vi "SWITCH Message Loop.vi"(8 "error in (no error)":errorcluster) -> (0 "error out":errorcluster)   [LabVIEW 2020, in "MOTOR.lvlib"]
doc: "Message loop for handling messages pertaining to the acquisition of data from the hardware."
uses:
  MOTOR.lvlib
  support/PCT FGV CMD.ctl
  Acquisition State.ctl
  PS Hardware Configuration.ctl
  support/Message Queue/Message Cluster.ctl
  support/Message Queue/Enqueue Message (Single).vi
  <vilib>/Utility/error.llb/Error Cluster From Error Code.vi
  <vilib>/ErrorRing/Error Ring.xnode
  support/Message Queue/Message Queue.lvlib
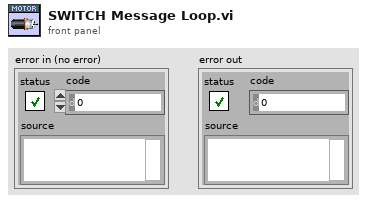
[diagram p1: front panel]
types:
  T1 = typedef "PCT FGV CMD.ctl" = enum16{"INIT", "GET", "SET"}
  T2 = typedef "Message Queue.lvlib/All Message Queues.ctl" = cluster{"UI":refnum<queue>, "Logging":refnum<queue>, "LOG":refnum<queue>, "ALARM":refnum<queue>, "Test":refnum<queue>, "Answer":refnum<queue>, "PLC":refnum<queue>, "DB":refnum<queue>, "Report":refnum<queue>, "OPC":refnum<queue>, "Procedure":refnum<queue>, "PalmSens":refnum<queue>, "SYS 7000 Reader":refnum<queue>, "SWITCH":refnum<queue>, "MOTOR":refnum<queue>, "MOTION":refnum<queue>, "HIDEN":refnum<queue>, "VALVE":refnum<queue>, "MFC":refnum<queue>, "PUMP IN":refnum<queue>, "PUMP OUT":refnum<queue>}
  T3 = typedef "PCT Data REFs.ctl" = cluster{"PLC AI Notifier":refnum<notifier>, "PS Data Queue":refnum<queue>, "BTN Queue":refnum<queue>, "PLC DI notifier":refnum<notifier>, "Timer notifier":refnum<notifier>, "DMM PS":refnum<notifier>, "DMM Gages":refnum<notifier>, "XYZ notifier":refnum<notifier>, "Test Notifier":refnum<notifier>, "Scanner notifier":refnum<notifier>, "OPC Notifier":refnum<notifier>, "HIDEN queue":refnum<queue>}
  T4 = typedef "MOTOR.lvlib/PS Hardware Configuration.ctl" = cluster{"Tango HW":cluster{"VISA resource":refnum<visa-resource-name>, "Baud Rate (115200)":i32, "lAnInterfaceType":i32, "bAShowProt":i32}, "Writer Queue":refnum<queue>, "Status":bool, "Abs Position":i32[], "Axis Velocity":cluster{"dX":dbl, "dY":dbl, "dZ":dbl, "dA":dbl}, "acceleration ":dbl, "Z direction":enum16{"Up", "Down"}, "Position Mode":string, "plLSID":i32}
  T5 = typedef "Message Queue.lvlib/Message Cluster.ctl" = cluster{"Message":string, "Message Data":variant}
  T6 = typedef "MOTOR.lvlib/Acquisition State.ctl" = enum16{"Idle", "Initialized"}
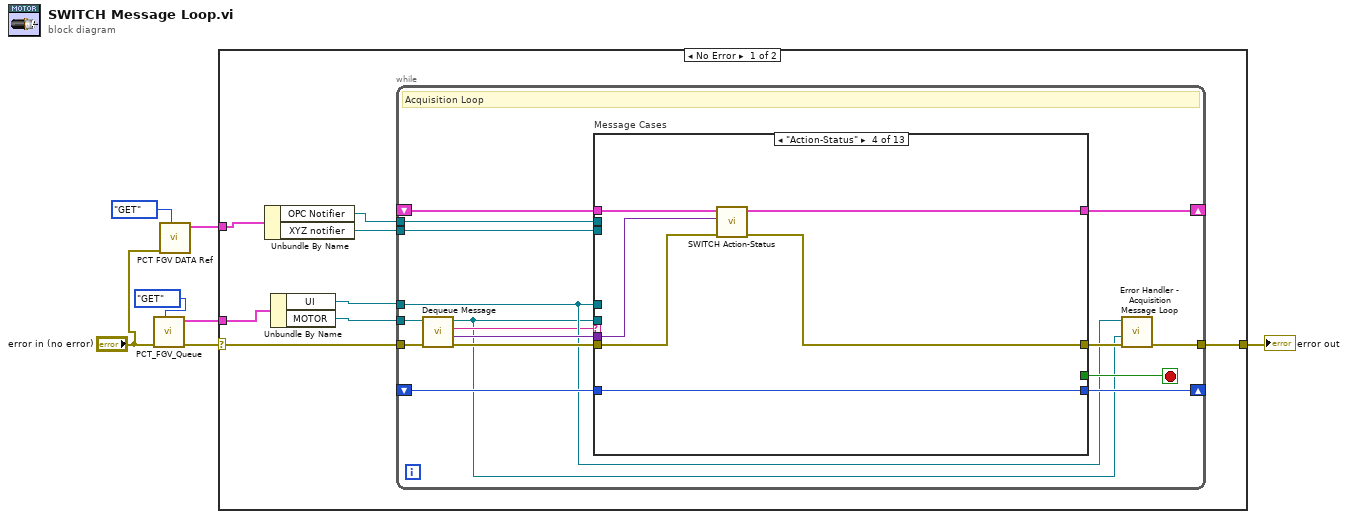
[diagram p0: block diagram]
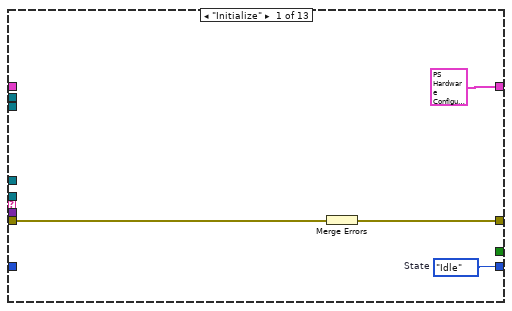
[diagram p2: hidden frame]
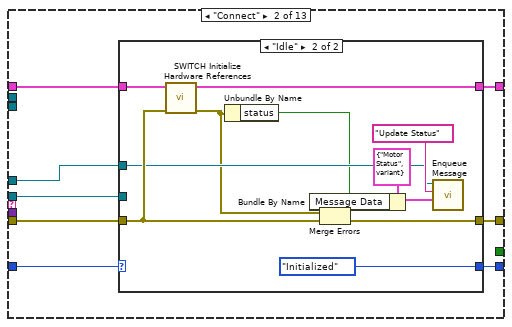
[diagram p3: hidden frame]
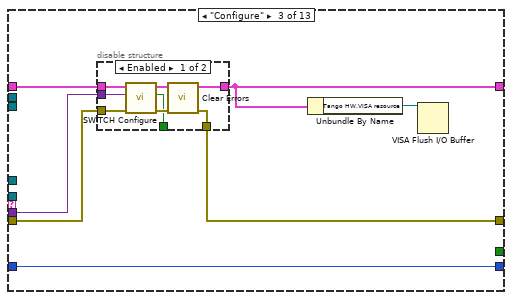
[diagram p5: hidden frame]
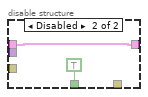
[diagram p6: hidden frame]
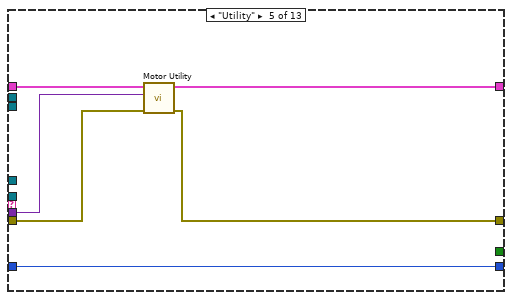
[diagram p7: hidden frame]
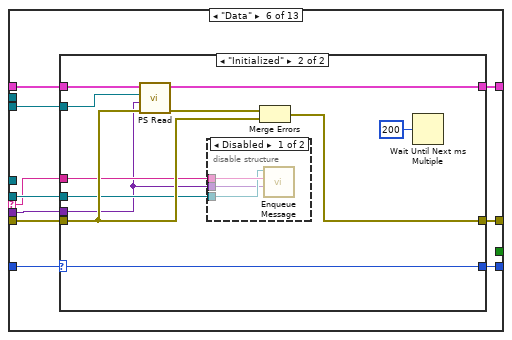
[diagram p8: hidden frame]
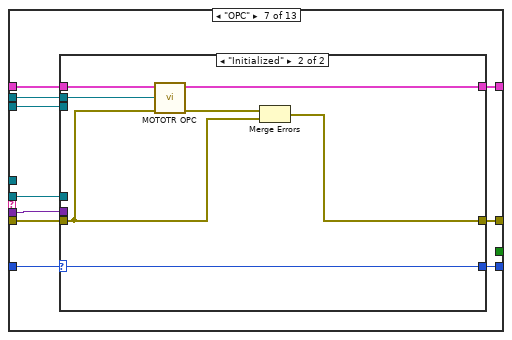
[diagram p11: hidden frame]
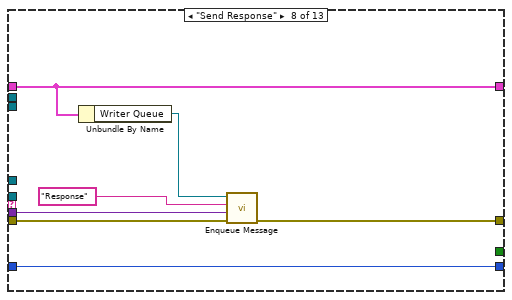
[diagram p13: hidden frame]
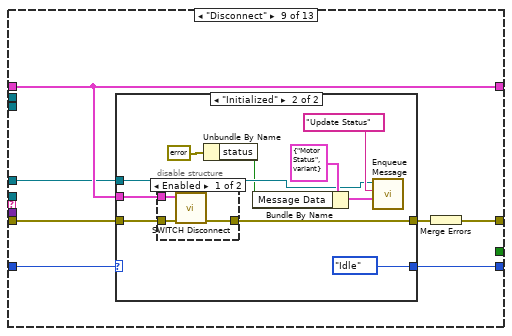
[diagram p14: hidden frame]
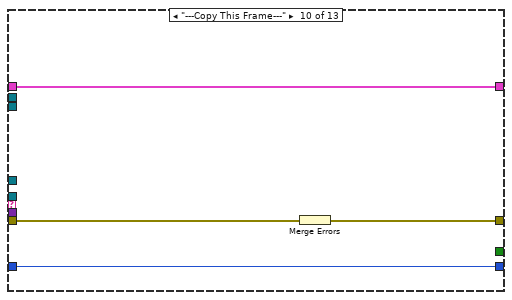
[diagram p17: hidden frame]
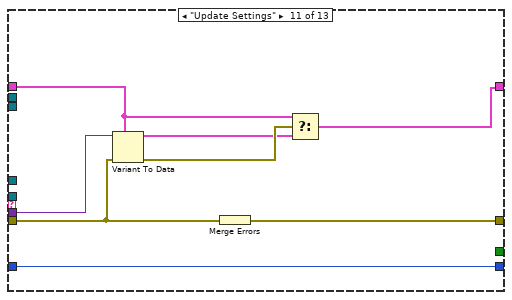
[diagram p18: hidden frame]
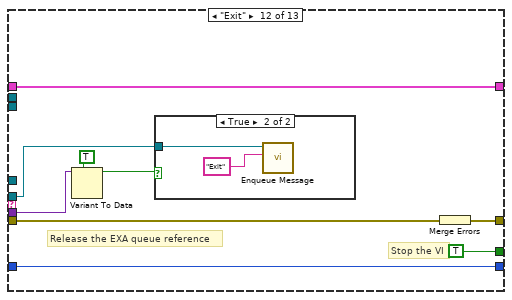
[diagram p19: hidden frame]
diagram:
  n1 = call "PCT_FGV_Queue.vi"("CMD"=PCT_FGV_CMD."GET", "error in (no error)"="error in (no error)") -> ("error out"=w5:errorcluster, "Message Queues out"=w4:T2)  [unwired: 8 in]
  n2 = call "PCT FGV DATA Ref.vi"("CMD"=PCT_FGV_CMD."GET", "error in (no error)"="error in (no error)") -> ("Data REF"=w1:T3)  [unwired: 8 in, 1 out]
  n3 = case shown="No Error" w5 {
    selector: w5 -> [w12 w196]
    tunnel: w4 -> [w15 _]
    tunnel: [w13 w196] -> w7
    tunnel: w1 -> [w10 _]
    frame No Error {
      n4 = Unbundle By Name(w10) -> ("OPC Notifier"=w8:refnum<notifier>, "XYZ notifier"=w9:refnum<notifier>)
      n5 = Unbundle By Name(w15) -> ("UI"=w11:refnum<queue>, "MOTOR"=w14:refnum<queue>)
      n6 = while {
        tunnel: w14 -> [w25]
        shift-right: [w30] -> _
        shift-left: _ -> [w31]
        tunnel: w11 -> [w20]
        shift-right: [w23] -> _
        shift-left: _ -> [w24]
        tunnel: w12 -> [w28]
        tunnel: [w22] -> w13
        tunnel: w9 -> [w18]
        tunnel: w8 -> [w16]
        stop <- w29 stop-if-true
        # "Acquisition Loop"
        n7 = call "Dequeue Message.vi"("error in (no error)"=w28, "Message Queue"=w25) -> ("error out"=w27:errorcluster, "Message Data"=w26:variant, "Message"=w19:string, "dup Message Queue"=w17:refnum<queue>)  [unwired: 6 in]
        n8 = case "Message Cases" shown="\"Action-Status\"" w19 {
          selector: w19 -> [_ _ _ _ _ w86 _ _ _ _ _ _ w185]
          tunnel: w17 -> [_ w40 _ _ _ w94 w121 _ _ _ _ w176 _]
          tunnel: w27 -> [w34 w41 w61 w75 w82 w93 w120 w137 w145 w165 w167 w175 _]
          tunnel: [w35 w43 w60 w74 w80 w95 w122 w136 w146 w163 w173 w181 w186] -> w21
          tunnel: w31 -> [_ w42 w62 w76 w84 w91 w118 w134 w143 w164 w169 w180 w188]
          tunnel: [T4 {"Tango HW"={"VISA resource"="", "Baud Rate (115200)"=0, "lAnInterfaceType"=0, "bAShowProt"=2}, "Writer Queue"=refnum, "Status"=FALSE, "Abs Position"=[], "Axis Velocity"={"dX"=0.0, "dY"=0.0, "dZ"=0.0, "dA"=0.0}, "acceleration "=0.0, "Z direction"=enum."Up", "Position Mode"="", "plLSID"=0} ("Data Cluster") w39 w59 w77 w81 w92 w119 w134 w143 w164 w168 w180 w188] -> w30
          tunnel: [_ _ _ _ _ _ _ _ _ _ _ TRUE _] -> w29
          tunnel: w26 -> [_ _ w63 w78 w83 w88 w115 w135 _ _ w172 w174 _]
          tunnel: w20 -> [_ w36 _ _ _ _ _ _ w140 _ _ _ _]
          tunnel: w24 -> [_ w37 w64 w79 w85 w89 w116 w138 w142 w162 w166 w179 w187]
          tunnel: [w33 w38 w64 w79 w85 w90 w117 w138 w141 w162 w166 w179 w187] -> w23
          tunnel: w18 -> [_ _ _ _ _ w87 w114 _ _ _ _ _ _]
          tunnel: w16 -> [_ _ _ _ _ _ w113 _ _ _ _ _ _]
          frame "Initialize" {
            w33 = Acquisition_State."Idle"  # State
            # "Initialize  - Initialize is currently a no-op.  The hardware initialization takes place in the 'Start' message."
            n9 = Merge Errors(w34) -> (w35:errorcluster)
          }
          frame "Connect" {
            # "Start - Configure and start the acquisition."
            n10 = case shown="\"Idle\"" w37 {
              selector: w37 -> [w44 _]
              tunnel: [w45 w57] -> w43
              tunnel: w42 -> [w46 w56]
              tunnel: w41 -> [w45 w53]
              tunnel: w40 -> [_ _]
              tunnel: [w46 w55] -> w39
              tunnel: [w44 Acquisition_State."Initialized" ("Acquisition State")] -> w38
              tunnel: w36 -> [_ w49]
              frame "Initialized" {
                # "The system is already acquiring. Ignore the \"Start\" message."
              }
              frame "Idle" {
                # "If the system is idle, start the acquisition."
                n11 = call "SWITCH Initialize Hardware References.vi"("error in (no error)"=w53, "Hardware Resources in"=w56) -> ("error out"=w48:errorcluster, "Hardware Resources out"=w55:T4)  [unwired: 8 in]
                n12 = Unbundle By Name(w48) -> ("status"=w47:bool)
                n13 = Bundle By Name(cluster=T5 {"Message"="Motor Status", "Message Data"=variant} ("Message Cluster"), "Message Data"=w47) -> (w51:T5)
                n14 = Merge Errors(w48, w53) -> (w57:errorcluster)
                n15 = call-poly "Enqueue Message.vi"("Message Data"=w51, "Message"="Update Status", "Message Queue"=w49) -> ()  [unwired: 7 in, 2 out]
              }
            }
          }
          frame "Configure" {
            # "Start - Configure and start the acquisition."
            n16 = disable-structure shown="Enabled" {
              disable-tunnel: w63 -> [w71 _]
              disable-tunnel: w62 -> [w70 w73]
              disable-tunnel: w61 -> [w69 _]
              disable-tunnel: [w67 w73] -> w59
              disable-tunnel: [w66 _] -> w60
              disable-tunnel: [w65 TRUE ("Send Resp")] -> _
              frame Enabled {
                n17 = call "SWITCH Configure.vi"("error in (no error)"=w69, "Message Data"=w71, "Data Cluster"=w70) -> ("error out"=w68:errorcluster, "Send Resp"=w65:bool, "Data Cluster out"=w67:T4)  [unwired: 6 in]
                n18 = call <vilib>:"Clear Errors.vi"("error in (no error)"=w68) -> ("error out"=w66:errorcluster)  [unwired: 5 in, 1 out]
              }
              frame Disabled {
              }
            }
            n19 = Unbundle By Name(w59) -> ("Tango HW.VISA resource"=w58:refnum<visa-resource-name>)
            n20 = VISA Flush I/O Buffer(VISA resource name=w58) -> ()  [unwired: 2 in, 2 out]
          }
          frame "Action-Status" {
            # "Start - Configure and start the acquisition."
            n21 = call "SWITCH Action-Status.vi"("error in (no error)"=w75, "Message Data"=w78, "Data Cluster"=w76) -> ("error out"=w74:errorcluster, "Data Cluster out"=w77:T4)  [unwired: 7 in]
          }
          frame "Utility" {
            # "Start - Configure and start the acquisition."
            n22 = call "Motor Utility.vi"("error in (no error)"=w82, "Message Data"=w83, "Data Cluster"=w84) -> ("error out"=w80:errorcluster, "Data Cluster out"=w81:T4)  [unwired: 7 in]
          }
          frame "Data" {
            # "Acquire - Acquire data from the hardware. Since this is a continuous acquisition, this message will always message itself to run again."
            n23 = case shown="\"Initialized\"" w89 {
              selector: w89 -> [w96 w105]
              tunnel: [w97 w109] -> w95
              tunnel: w94 -> [_ w101]
              tunnel: w93 -> [w97 w103]
              tunnel: [w98 w107] -> w92
              tunnel: w91 -> [w98 w106]
              tunnel: [w96 w105] -> w90
              tunnel: w88 -> [_ w99]
              tunnel: w87 -> [_ w104]
              tunnel: w86 -> [_ w102]
              frame "Idle" {
              }
              frame "Initialized" {
                # "Read  data"
                n24 = call "PS Read.vi"("error in (no error)"=w103, "Message Data"=w99, "XYZ notifier"=w104, "Hardware Resources in"=w106) -> ("error out"=w108:errorcluster, "Hardware Resources out"=w107:T4)  [unwired: 5 in, 1 out]
                n25 = disable-structure shown="Disabled" {
                  disable-tunnel: w102 -> [w112 _]
                  disable-tunnel: w101 -> [w111 _]
                  disable-tunnel: w99 -> [w110 _]
                  frame Disabled {
                    n26 = call-poly "Enqueue Message.vi"("Message Data"=w110, "Message"=w112, "Message Queue"=w111) -> ()  [unwired: 7 in, 2 out]
                  }
                  frame Enabled {
                  }
                }
                n27 = Merge Errors(w108, w103) -> (w109:errorcluster)
                n28 = Wait Until Next ms Multiple(millisecond multiple=u32 200) -> ()  [unwired: 1 out]
              }
            }
          }
          frame "OPC" {
            # "Acquire - Acquire data from the hardware. Since this is a continuous acquisition, this message will always message itself to run again."
            n29 = case shown="\"Initialized\"" w116 {
              selector: w116 -> [w123 w131]
              tunnel: [w124 w132] -> w122
              tunnel: w121 -> [_ _]
              tunnel: w120 -> [w124 w128]
              tunnel: [w125 w129] -> w119
              tunnel: w118 -> [w125 w130]
              tunnel: [w123 w131] -> w117
              tunnel: w115 -> [_ _]
              tunnel: w114 -> [_ _]
              tunnel: w113 -> [_ w126]
              frame "Idle" {
              }
              frame "Initialized" {
                # "Read  data"
                n30 = call "MOTOTR OPC.vi"("error in (no error)"=w128, "OPC Notifier"=w126, "Hardware Resources in"=w130) -> ("error out"=w127:errorcluster, "Hardware Resources out"=w129:T4)  [unwired: 7 in]
                n31 = Merge Errors(w127, w128) -> (w132:errorcluster)
              }
            }
          }
          frame "Send Response" {
            # "Acquire - Acquire data from the hardware. Since this is a continuous acquisition, this message will always message itself to run again."
            n32 = Unbundle By Name(w134) -> ("Writer Queue"=w133:refnum<queue>)
            n33 = call-poly "Enqueue Message.vi"("error in (no error)"=w137, "Message Data"=w135, "Message"="Response", "Message Queue"=w133) -> ("error out"=w136:errorcluster)  [unwired: 6 in, 1 out]
          }
          frame "Disconnect" {
            # "Stop - Stop the Acquisition."
            n34 = case shown="\"Initialized\"" w142 {
              selector: w142 -> [w147 _]
              tunnel: w145 -> [w148 w158]
              tunnel: [w148 w157] -> w144
              tunnel: w143 -> [_ w156]
              tunnel: [w147 Acquisition_State."Idle" ("State")] -> w141
              tunnel: w140 -> [_ w150]
              frame "Idle" {
                # "The system is already idle. Ignore the \"Stop\" message."
              }
              frame "Initialized" {
                # "If the system is acquiring, stop the acquisition."
                n35 = disable-structure shown="Enabled" {
                  disable-tunnel: w158 -> [w161 _]
                  disable-tunnel: [w160 _] -> w157
                  disable-tunnel: w156 -> [w159 _]
                  frame Enabled {
                    n36 = call "SWITCH Disconnect.vi"("error in (no error)"=w161, "Hardware Resources in"=w159) -> ("error out"=w160:errorcluster)  [unwired: 9 in]
                  }
                  frame Disabled {
                  }
                }
                n37 = Unbundle By Name(errorcluster {"status"=TRUE, "code"=6001, "source"=""} ("error out")) -> ("status"=w149:bool)
                n38 = Bundle By Name(cluster=T5 {"Message"="Motor Status", "Message Data"=variant} ("Message Cluster"), "Message Data"=w149) -> (w153:T5)
                n39 = call-poly "Enqueue Message.vi"("Message Data"=w153, "Message"="Update Status", "Message Queue"=w150) -> ()  [unwired: 7 in, 2 out]
              }
            }
            n40 = Merge Errors(w144) -> (w146:errorcluster)
          }
          frame "---Copy This Frame---" {
            # "Duplicate this frame when creating new messages.  Change this comment in the duplicated frame to describe this message."
            n41 = Merge Errors(w165) -> (w163:errorcluster)
          }
          frame "Update Settings" {
            # "New settings are available, update the current ones stored in the shift register with the settings sent as part of the message"
            n42 = Variant To Data(error in=w167, type=w169, Variant=w172) -> (data=w170:T4, error out=w171:errorcluster)
            n43 = Merge Errors(w167) -> (w173:errorcluster)
            n44 = Select(t=w169, s=w171, f=w170) -> (s? t:f=w168:T4)
          }
          frame "Exit" {
            # "Release the EXA queue reference"
            # "Stop the VI"
            # "Exit - Send the Exit message to the UI Message Handler."
            n45 = Variant To Data(type=TRUE, Variant=w174) -> (data=w178:bool)  [unwired: 1 in, 1 out]
            n46 = case shown="True" w178 {
              tunnel: w176 -> [_ w184]
              frame False {
              }
              frame True {
                n47 = call-poly "Enqueue Message.vi"("Message"="Exit", "Message Queue"=w184) -> ()  [unwired: 8 in, 2 out]
              }
            }
            n48 = Merge Errors(w175) -> (w181:errorcluster)
          }
          frame Default {
            # "'Default' case only runs if there is a message that isn't defined in any of the other cases.  Output a programming error."
            n49 = xnode "Error Ring"("parameter 0"=w185) -> ("error out"=w186:errorcluster)
          }
        }
        n50 = call "Error Handler - Acquisition Message Loop.vi"("error in (no error)"=w21, "Motor"=w17, "Message Queue"=w20) -> ("dup error in"=w22:errorcluster)  [unwired: 7 in, 1 out]
      }
    }
    frame Error {
    }
  }
  "error out" <- w7
